vi "Upate Step Num Indicator From Ref.vi"(8 "Error In":errorcluster, 9 "Active Step Display Ref":refnum<vi>, 10 "Recorded Data Buffer Ref":refnum<vi>, 11 "Active Step Num Ref":refnum<vi>) -> (0 "Error Out":errorcluster)   [LabVIEW 2017]
doc: "This VI updates step number in the following format: \"%d of %d\"\n\nParams: \nuint8_t* Active Step Num Ref -> formatted to first &d\nuint64_t Recorded Data Buffer Ref [] -> length formatted to second %d\nstring* Active Step Display Ref -> string to output data to"
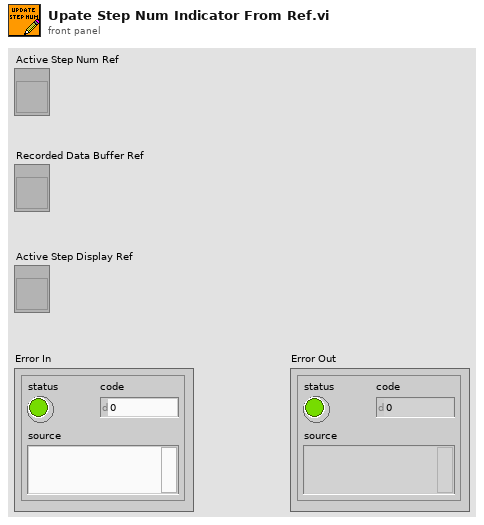
[diagram p1: front panel]
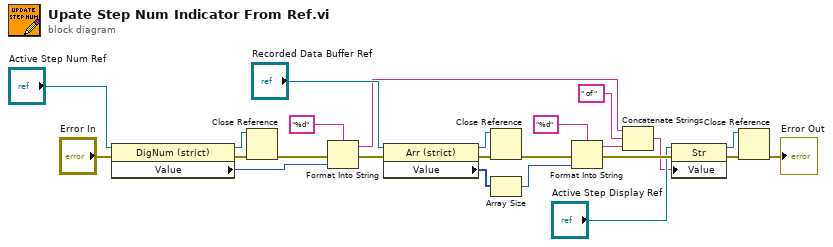
[diagram p0: block diagram]
diagram:
  n1 = property class="DigNum (strict)"(reference="Active Step Num Ref", error in="Error In") -> (reference out=w19:refnum<vi>, error out=w20:errorcluster, "Value"=w21:u8)
  n2 = Close Reference(reference=w19, error in (no error)=w20) -> (error out=w18:errorcluster)
  n3 = Format Into String(format string="%d", error in=w18, w21) -> (resulting string=w7:string, error out=w17:errorcluster)  [unwired: 1 in]
  n4 = property class="Arr (strict)"(reference="Recorded Data Buffer Ref", error in=w17) -> (reference out=w14:refnum<vi>, error out=w15:errorcluster, "Value"=w13:u64[])
  n5 = Close Reference(reference=w14, error in (no error)=w15) -> (error out=w10:errorcluster)
  n6 = Array Size(array=w13) -> (size(s)=w11:i32)
  n7 = Format Into String(format string="%d", error in=w10, w11) -> (resulting string=w8:string, error out=w6:errorcluster)  [unwired: 1 in]
  n8 = Concatenate Strings(w7, " of " ("string"), w8) -> (w4:string)
  n9 = property class="Str"(reference="Active Step Display Ref", error in=w6, "Value"=w4) -> (reference out=w2:refnum<vi>, error out=w3:errorcluster)
  n10 = Close Reference(reference=w2, error in (no error)=w3) -> (error out=→"Error Out":errorcluster)
